vi "Przełącznik D.vi"(9 "R":bool, 10 "C":bool, 11 "D":bool) -> (2 "~Q":bool, 3 "Q":bool)   [LabVIEW 2020]
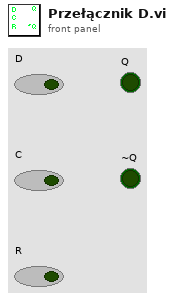
[diagram p1: front panel]
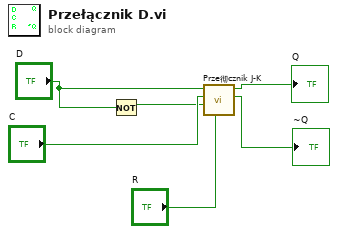
[diagram p0: block diagram]
diagram:
  n1 = Not(x="D") -> (.not. x?=w1:bool)
  n2 = call "Prze彻cznik J-K.vi"("R"="R", "K"=w1, "C"="C", "J"="D") -> ("~Q"=→"~Q":bool, "Q"=→"Q":bool)  [unwired: 6 in]
